vi "Read_temp_to_file.vi"() -> ()   [LabVIEW 2017]
uses:
  <instrlib>/Lake Shore 336/Public/Data/Sensor Data (Single Reading).vi
  <vilib>/Utility/file.llb/Write Delimited Spreadsheet (DBL).vi
  <instrlib>/Lake Shore 336/Lake Shore 336.lvlib
panel:
  in  "Save or not":bool
  in  "file path (dialog if empty)":path
  in  "precision (6)":i16
  in  "width (-)":i16
  out "Temperature":string
  in  "Input (0:A)":u16(ring) items=["A", "B", "C", "D"]
  in  "Data Source (0:Kelvin)":u16(ring) items=["Kelvin", "Celsius", "Sensor Units"]
  in  "Serial Configuration":T1={"Baud Rate"=57600, "Parity"=1, "Data Bits"=7, "Stop Bits"=10, "Flow Control"=0} {"Flow Control" items=["None", "XON/XOFF", "RTS/CTS", "XON/XOFF & RTS/CTS", "DTR/DSR", "XON/XOFF & DTR/DSR"]; "Stop Bits" items=["1.0"=10, "1.5"=15, "2.0"=20]; "Data Bits" items=["7"=7, "8"=8]; "Parity" items=["None", "Odd", "Even", "Mark", "Space"]; "Baud Rate" items=["300"=300, "600"=600, "1200"=1200, "2400"=2400, "4800"=4800, "9600"=9600, "19200"=19200, "38400"=38400, "57600"=57600]}
  in  "VISA resource name":refnum<visa-resource-name>
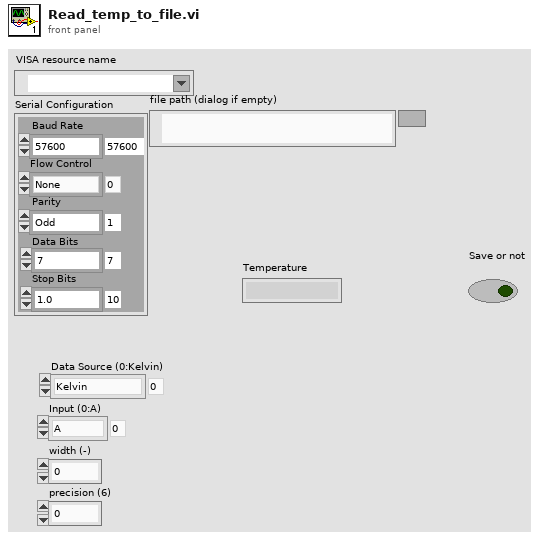
[diagram p1: front panel]
types:
  T1 = cluster{"Baud Rate":u32, "Parity":u16, "Data Bits":u16, "Stop Bits":u16, "Flow Control":u16}
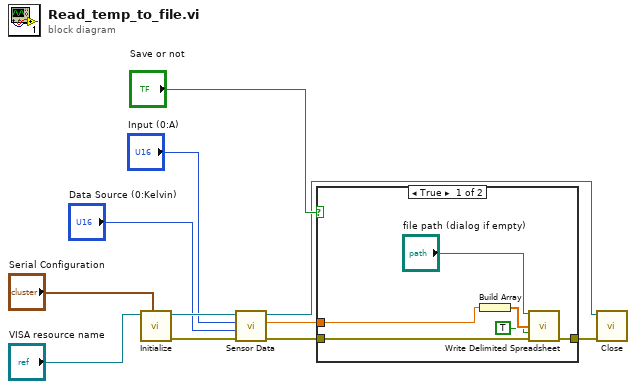
[diagram p0: block diagram]
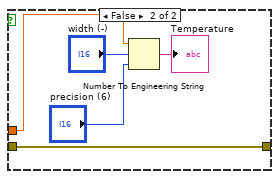
[diagram p2: hidden frame]
diagram:
  n1 = call <instrlib>:"Initialize.vi"("Serial Configuration"="Serial Configuration", "VISA resource name"="VISA resource name") -> ("error out"=w6:errorcluster, "VISA resource name out"=w9:refnum<visa-resource-name>)  [unwired: 8 in]
  n2 = call-poly <instrlib>:"Sensor Data.vi"("error in (no error)"=w6, "Data Source (0:Kelvin)"="Data Source (0:Kelvin)", "Input (0:A)"="Input (0:A)", "VISA resource name"=w9) -> ("error out"=w2:errorcluster, "Sensor Data"=w5:dbl, "VISA resource name out"=w3:refnum<visa-resource-name>)  [unwired: 5 in]
  n3 = case shown="True" "Save or not" {
    tunnel: w5 -> [w16 w19]
    tunnel: w2 -> [w13 w18]
    tunnel: [w12 w18] -> w1
    frame True {
      n4 = Build Array(w16) -> (w15:dbl[])
      n5 = call-poly <vilib>:"Write Delimited Spreadsheet.vi"("file path (dialog if empty)"="file path (dialog if empty)", "1D data"=w15, "append to file? (new file:F)"=TRUE, "error in (no error)"=w13) -> ("error out"=w12:errorcluster)  [unwired: 10 in, 1 out]
    }
    frame False {
      n6 = Number To Engineering String(2:"precision (6)", 3:"width (-)", 4:w19) -> (0:→"Temperature":string)  [unwired: 1 in]
    }
  }
  n7 = call <instrlib>:"Close.vi"("error in (no error)"=w1, "VISA resource name"=w3) -> ()  [unwired: 9 in, 1 out]
